vi "FGV Autokal GT.vi"(6 "Aktion FGV AutoKal":T1, 8 "error in (no error)":errorcluster caption="Fehler (Eingang, kein Fehler)", 10 "Start LinCheck":refnum<vi>, 11 "Autokal GT Aktiv?":bool) -> (0 "error out":errorcluster caption="Fehler (Ausgang)", 2 "Start LinCheck":refnum<vi>, 3 "Autokal GT Aktiv?":bool)   [LabVIEW 2020, in "Auto Kalibrieren.lvlib"]
uses:
  Auto Kalibrieren.lvlib
  Aktion FGV Autokal GT.ctl
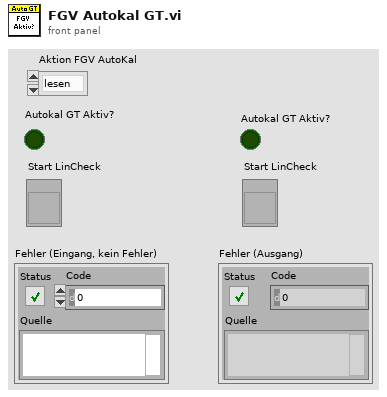
[diagram p1: front panel]
types:
  T1 = typedef "Auto Kalibrieren.lvlib/Aktion FGV Autokal GT.ctl" = enum16{"lesen", "Autokal GT", "Referenz Start"}
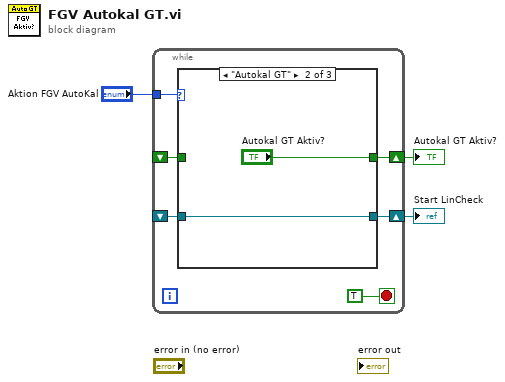
[diagram p0: block diagram]
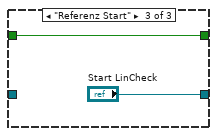
[diagram p3: hidden frame]
diagram:
  n1 = while {
    tunnel: "Aktion FGV AutoKal" -> [w8]
    shift-right: [w7] -> w2
    shift-left: _ -> [w6]
    shift-right: [w5] -> w1
    shift-left: _ -> [w4]
    stop <- TRUE stop-if-true
    n2 = case shown="\"Autokal GT\"" w8 {
      tunnel: [w11 "Autokal GT Aktiv?" w15] -> w7
      tunnel: w6 -> [w11 _ w15]
      tunnel: [w10 w12 "Start LinCheck"] -> w5
      tunnel: w4 -> [w10 w12 _]
      frame "lesen", Default {
      }
      frame "Autokal GT" {
      }
      frame "Referenz Start" {
      }
    }
  }
  "Autokal GT Aktiv?" <- w2
  "Start LinCheck" <- w1
